vi "S2C_VAR_AddToDB.vi"(8 "Error In":errorcluster) -> (0 "Error Out":errorcluster)   [LabVIEW 2015]
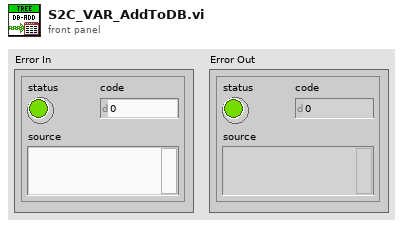
[diagram p1: front panel]
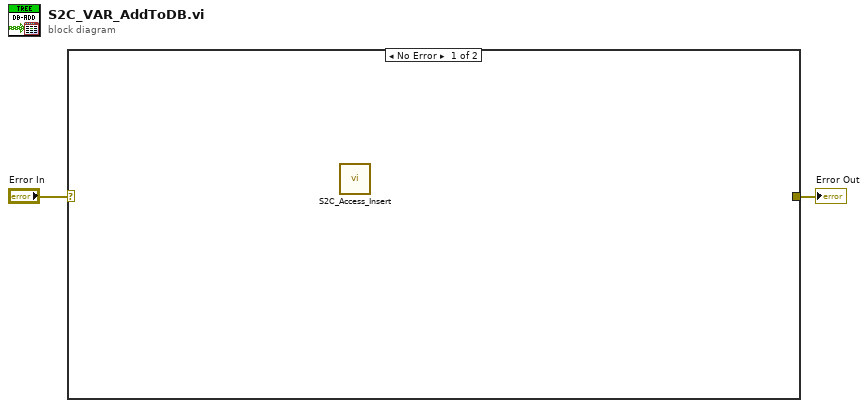
[diagram p0: block diagram]
diagram:
  n1 = case shown="No Error" "Error In" {
    selector: "Error In" -> [_ w4]
    tunnel: [w3 w4] -> w1
    frame No Error {
      n2 = call "S2C_Access_Insert.vi"() -> ()  [unwired: 11 in, 1 out]
    }
    frame Error {
    }
  }
  "Error Out" <- w1
